vi "Decode ICMP Packet.vi"(11 "ICMP Packet":u8[](array[numeric]) format="%02x") -> (2 "Valid Packet?":bool, 3 "ICMP Packet Info":T1 {"Sequence Number" format="%04x"; "ID" format="%04x"; "Checksum" format="%04x"; "Data" format="%02x"})   [LabVIEW 2018]
uses:
  ICMP Packet Info.ctl
panel:
  out "cksum (U16)":u16 format="%04x"
  # "U8"
  # "U8"
  # "U16"
  # "U16"
  # "U16"
  # "U32"
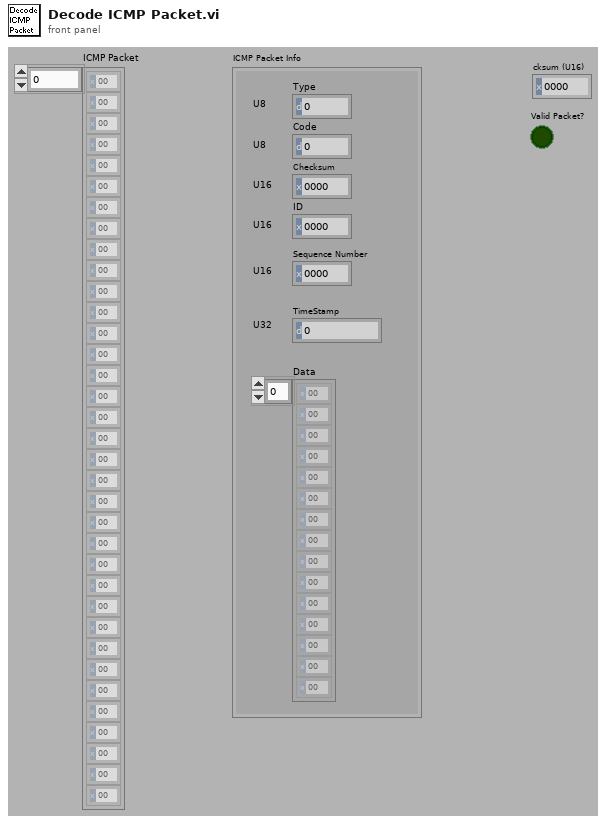
[diagram p1: front panel]
types:
  T1 = typedef "ICMP Packet Info.ctl" = cluster{"Type":u8, "Code":u8, "Checksum":u16, "ID":u16, "Sequence Number":u16, "TimeStamp":u32, "Data":u8[]}
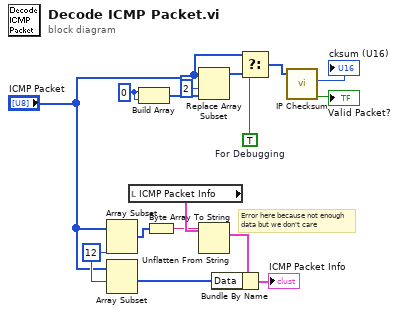
[diagram p0: block diagram]
diagram:
  w5 = 12 ("length")
  w10 = TRUE  # For Debugging
  w14 = u8 0 ("index")
  # "Error here because not enough\ndata but we don't care"
  n1 = Array Subset(array="ICMP Packet", length=w5) -> (w6:u8[])  [unwired: 1 in]
  n2 = Array Subset(array="ICMP Packet", index=w5) -> (w1:u8[])  [unwired: 1 in]
  n3 = local read "ICMP Packet Info"() -> (w8:T1)
  n4 = Build Array(w14, w14) -> (w9:u8[])
  n5 = Byte Array To String(unsigned byte array=w6) -> (string=w7:string)
  n6 = Replace Array Subset(array="ICMP Packet", new element=w9, index=2) -> (w11:u8[])
  n7 = Unflatten From String(type=w8, binary string=w7) -> (value=w4:T1)  [unwired: 3 in, 2 out]
  n8 = Bundle By Name(cluster=w4, "Data"=w1) -> (→"ICMP Packet Info":T1)
  n9 = Select(t="ICMP Packet", s=w10, f=w11) -> (s? t:f=w12:u8[])
  n10 = call "IP Checksum.vi"("Packet (U8)"=w12) -> ("Valid Packet?"=→"Valid Packet?":bool, "cksum (U16)"=→"cksum (U16)":u16)  [unwired: 7 in, 2 out]
